vi "Labview_FFT.vi"(0 "Channel A":u16[][](array[numeric]), 5 "Range":dbl format="%#_13g", 7 "Bits":dbl) -> (4 "Int B-Scan Channel A":sgl[][](array[numeric]))   [LabVIEW 2014]
uses:
  <vilib>/Analysis/4window.llb/Hanning Window (DBL).vi
  <vilib>/Analysis/2dsp.llb/Real FFT.vi
  <vilib>/Analysis/4window.llb/AllCosWindow (DBL).vi
  <vilib>/Analysis/NI_AALPro.lvlib
panel:
  in  "Log10?":bool
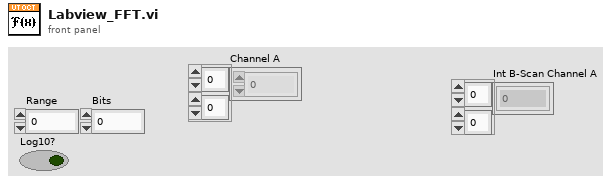
[diagram p1: front panel]
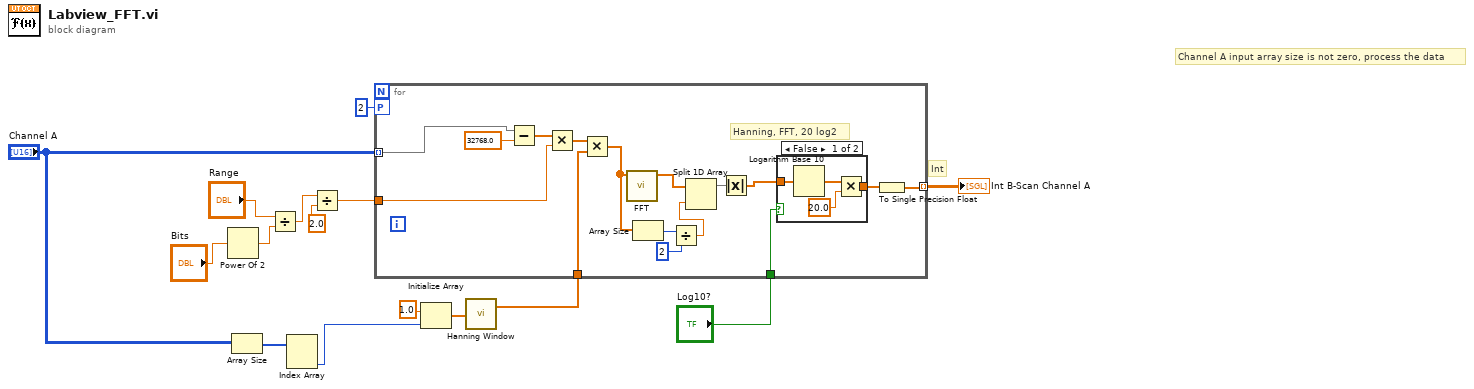
[diagram p0: block diagram]
diagram:
  # "Channel A input array size is not zero, process the data"
  # "Int"
  n1 = Power Of 2(x="Bits") -> (2^x=w15:dbl)
  n2 = Array Size(array="Channel A") -> (size(s)=w2:i32[])
  n3 = Divide(x="Range", y=w15) -> (x/y=w13:dbl)
  n4 = Index Array(array=w2) -> (element #2=w1:i32)  [unwired: 2 in, 1 out]
  n5 = Divide(x=w13, y=2.0) -> (x/y=w5:dbl)
  n6 = Initialize Array(1.0 ("element"), w1) -> (w11:dbl[])
  n7 = call-poly <vilib>:"Hanning Window.vi"("X"=w11) -> ("Windowed X"=w8:dbl[])  [unwired: 1 out]
  n8 = for {
    tunnel: [w18] -> w14 mode=indexing
    tunnel: w8 -> [w21]
    workers-P: 2 -> [_]
    tunnel: w5 -> [w20]
    tunnel: "Channel A" -> [w19] mode=indexing
    tunnel: "Log10?" -> [w16]
    # "Hanning, FFT, 20 log2"
    n9 = Subtract(x=w19, y=32768.0 ("element")) -> (x-y=w23:dbl[])
    n10 = Multiply(x=w23, y=w20) -> (x*y=w22:dbl[])
    n11 = Multiply(x=w22, y=w21) -> (x*y=w25:dbl[])
    n12 = call-poly <vilib>:"FFT.vi"("X"=w25) -> ("FFT {X}"=w27:cdb[])  [unwired: 9 in, 1 out]
    n13 = Array Size(array=w25) -> (size(s)=w31:i32)
    n14 = Divide(x=w31, y=2) -> (x/y=w29:dbl)
    n15 = Split 1D Array(array=w27, index=w29) -> (first subarray=w28:cdb[])  [unwired: 1 out]
    n16 = Absolute Value(x=w28) -> (abs(x)=w26:dbl[])
    n17 = case shown="False" w16 {
      tunnel: w26 -> [w35 w36]
      tunnel: [w32 w36] -> w17
      frame False {
        n18 = Logarithm Base 10(1:w35) -> (0:w34:dbl[])
        n19 = Multiply(x=w34, y=sgl 20.0) -> (x*y=w32:dbl[])
      }
      frame True {
      }
    }
    n20 = To Single Precision Float(number=w17) -> (single precision float=w18:sgl[])
  }
  "Int B-Scan Channel A" <- w14
